vi "Example HTTP POST method.vi"() -> ()   [LabVIEW 2015]
doc: "Example of using standard HTTP POST method with LabVIEW TCP/IP vi's to obtain data from ordinary web sites. Here posting means filling out a form and reading the resulting web page.\n\nThis typical example shows how posting a list of airports in ICAO format code to weather.noaa.gov gives the full METAR report of these airports (along with the full HTML source). The web site used here is http://weather.noaa.gov/weather/metar.shtml and the result is the same as manually inserting the airports in the form on that site. An automation of this POST method can be very useful for obtaining up to date background information (wind, temperature, polls etc) in connection with measurements, when collecting statistical data, or when sending measured data to a web site, just to mention a few uses. This method recieves the source HTML code in text format and does no attempt of displaying it in a browser like fashion (use the activeX webbrowser for that).\n\nA METAR report is an aronautical weather report (wind, visibility, humidity etc.) Try some other airports (must be 4 letter code according to the ICAO convention). This website will help you: http://www.ar-group.com/icaoiata.htm\n\nFor general information about the HTTP protocol and methods (POST, GET etc.) go to http://www.w3.org/Protocols\n\nBjornar Svingen\nbjornar.svingen@sintef.no bjornar.svingen@ktv.no"
panel:
  out "HTML source":string
  # "Example of using standard HTTP POST method with LabVIEW TCP/IP vi's to obtain data from ordinary web sites. Here posting means filling out a form and reading the resulting web page.\n\nThis typical example shows how posting a list of airports in ICAO format code to weather.noaa.gov gives the full METAR report of these airports (along with the full HTML source). The web site used here is http://weather.noaa.gov/weather/metar.shtml and the result is the same as manually inserting the airports in the form on that site. An automation of this POST method can be very useful for obtaining up to date background information (wind, temperature, polls etc) in connection with measurements, when collecting statistical data, or when sending measured data to a web site, just to mention a few uses. This method recieves the source HTML code in text format and does no attempt of displaying it in a browser like fashion (use the activeX webbrowser for that).\n\nA METAR report is an aronautical weather report (wind, visibility, humidity etc.) Try some other airports (must be 4 letter code according to the ICAO convention). This website will help you: http://www.ar-group.com/icaoiata.htm\n\nFor general information about the HTTP protocol and methods (POST, GET etc.) go to http://www.w3.org/Protocols\n\nBjornar Svingen\nbjornar.svingen@sintef.no   bjornar.svingen@ktv.no"
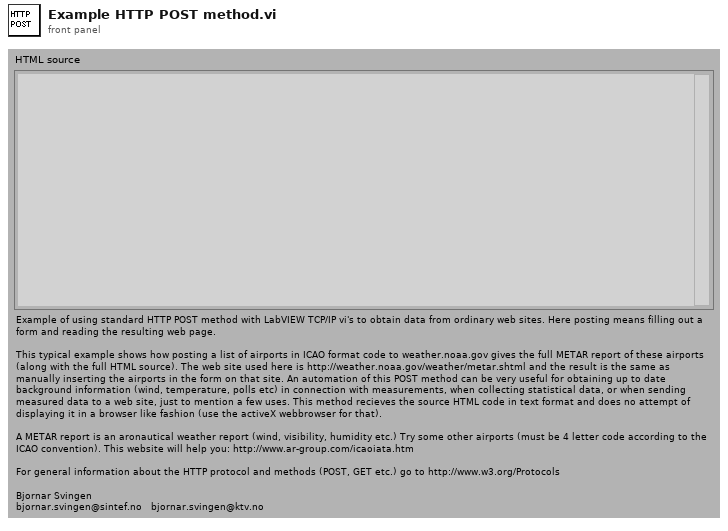
[diagram p1: front panel]
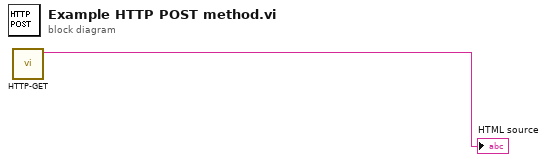
[diagram p0: block diagram]
diagram:
  n1 = call "HTTP-GET.vi"() -> ("String"=→"HTML source":string)  [unwired: 11 in]
